vi "VisibleControl.vi"() -> ()   [LabVIEW 2020]
panel:
  in  "Visible":bool
  in  "Numeric":dbl
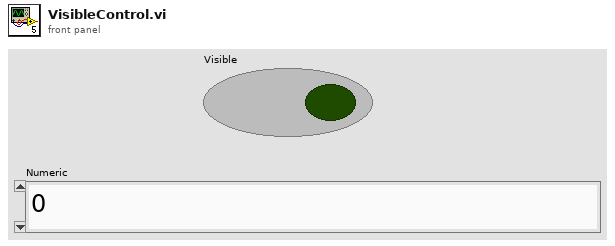
[diagram p1: front panel]
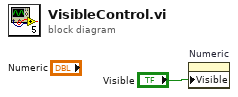
[diagram p0: block diagram]
diagram:
  n1 = property on="Numeric" class="DigNum (strict)"("Visible"="Visible") -> ()  [unwired: 2 in, 2 out]
